vi "XML_Get Tags by path.vi"(7 "delimiter (.)":string=".", 8 "error in (no error)":errorcluster, 10 "Tag path":string, 11 "XML String in":string) -> (0 "error out":errorcluster, 3 "Matching tag values":string[](array[string]))   [LabVIEW 2015, in "XML Parser.lvlib"]
uses:
  XML Parser.lvlib
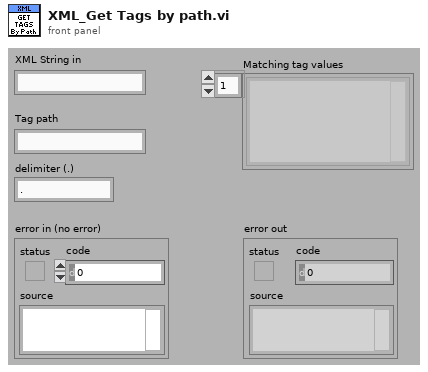
[diagram p1: front panel]
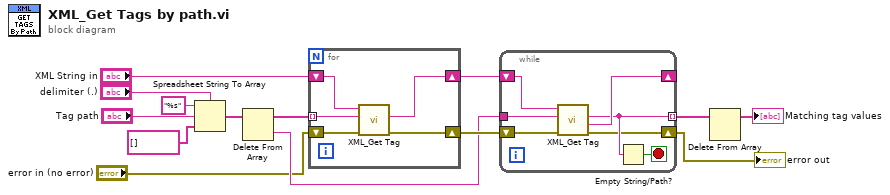
[diagram p0: block diagram]
diagram:
  n1 = Spreadsheet String To Array(delimiter (Tab)="delimiter (.)", format string="%s", spreadsheet string="Tag path", array type (2D Dbl)=string[] []) -> (array=w9:string[])
  n2 = Delete From Array(array=w9) -> (deleted portion=w5:string, array with subset deleted=w8:string[])  [unwired: 2 in]
  n3 = for {
    tunnel: w8 -> [w19] mode=indexing
    shift-right: [w15] -> w7
    shift-left: "XML String in" -> [w18]
    shift-right: [w16] -> w6
    shift-left: "error in (no error)" -> [w17]
    n4 = call "XML_Get Tag.vi"("error in (no error)"=w17, "Tag name"=w19, "XML String in"=w18) -> ("error out"=w16:errorcluster, "Tag value"=w15:string)  [unwired: 4 in, 3 out]
  }
  n5 = while {
    shift-right: [w23] -> _
    shift-left: w7 -> [w26]
    shift-right: [w20] -> w1
    shift-left: w6 -> [w25]
    tunnel: w5 -> [w24]
    tunnel: [w22] -> w4 mode=indexing
    stop <- w21 stop-if-true
    n6 = call "XML_Get Tag.vi"("error in (no error)"=w25, "Tag name"=w24, "XML String in"=w26) -> ("error out"=w20:errorcluster, "Remaining string"=w23:string, "Tag value"=w22:string)  [unwired: 4 in, 2 out]
    n7 = Empty String/Path?(string/path=w22) -> (empty?=w21:bool)
  }
  "error out" <- w1
  n8 = Delete From Array(array=w4) -> (array with subset deleted=→"Matching tag values":string[])  [unwired: 2 in, 1 out]
